vi "MdfInit.vi"(8 "error in (no error)":errorcluster, 9 "writer_type":i32(ring) items=["Mdf3Basic", "Mdf4Basic", "MdfBusLogger", "MdfConverter"], 11 "path_name":string) -> (0 "error out":errorcluster, 2 "Init":bool, 3 "MDFRef":refnum<k24>)   [LabVIEW 2025, in "MdfFile.lvlib"]
uses:
  MdfFile.lvlib
  data/mdflibrary.dll
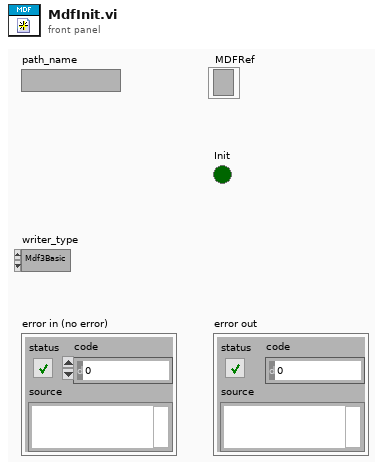
[diagram p1: front panel]
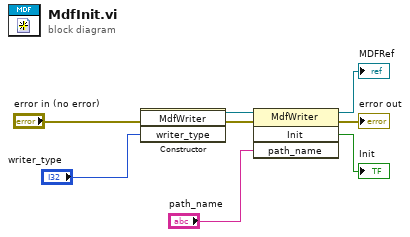
[diagram p0: block diagram]
diagram:
  n1 = constructor class="MdfWriter"(error in="error in (no error)", "writer_type"="writer_type") -> (reference out=w6:refnum<k24>, error out=w5:errorcluster)  [unwired: 2 in, 2 out]
  n2 = invoke class="MdfWriter" method="Init"(reference=w6, error in=w5, "path_name"="path_name") -> (reference out=→"MDFRef":refnum<k24>, error out=→"error out":errorcluster, "Init"=→"Init":bool)  [unwired: 1 in, 1 out]
